vi "Configure General Settings.vi"(1 "Jump Mode":u16(ring) items=["After Repetitions", "As soon as possible"], 2 "Wait Trigger on":u16(ring) items=["First Sample", "Last Sample"], 4 "Burst Selection":u16(ring) items=["Number of Cycles", "Default", "Minimum", "Maximum"], 5 "Burst Count":u32=1, 6 "Run Mode":u16(ring) items=["Continuous", "Single/Burst", "Triggered Continuous", "Stepped", "Advanced"], 7 "error in (no error)":errorcluster, 8 "Sample Decreasing Startegy":u16(ring) items=["Decimation", "Cut Tail", "Cut Head"], 9 "Sample Increasing Startegy":u16(ring) items=["Interpolation", "Return Zero", "Hold Last", "Samples Multiplication"], 10 "VISA resource name":refnum<visa-resource-name>) -> (0 "error out":errorcluster, 3 "VISA resource name out":refnum<visa-resource-name>)   [LabVIEW 2020, in "Active Technologies AWG3000.lvlib"]
uses:
  Active Technologies AWG3000.lvlib
panel:
  # "RESAMPLE STRATEGY"
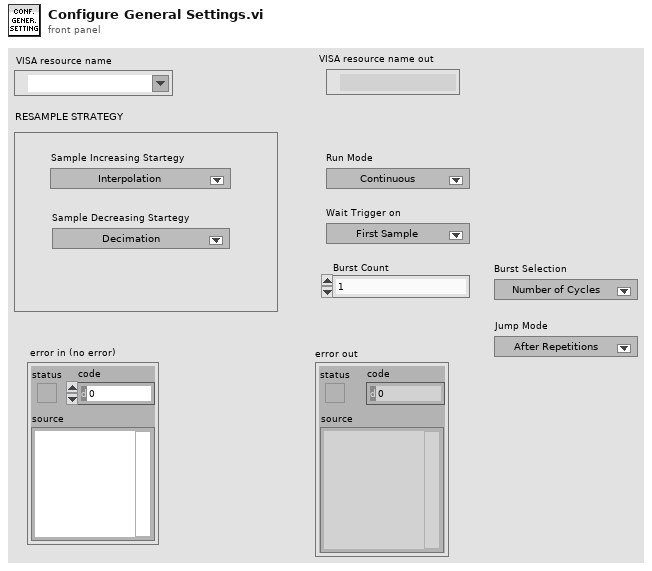
[diagram p1: front panel]
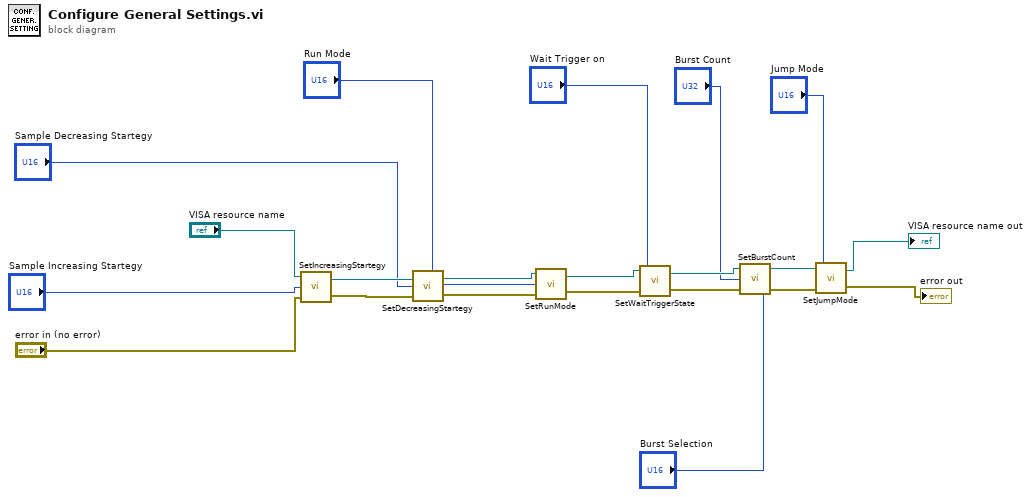
[diagram p0: block diagram]
diagram:
  n1 = call "SetIncreasingStartegy.vi"("error in (no error)"="error in (no error)", "Sample Increasing Startegy"="Sample Increasing Startegy", "VISA resource name"="VISA resource name") -> ("error out"=w16:errorcluster, "VISA resource name out"=w21:refnum<visa-resource-name>)
  n2 = call "SetDecreasingStartegy.vi"("error in (no error)"=w16, "Sample Decreasing Startegy"="Sample Decreasing Startegy", "VISA resource name"=w21) -> ("error out"=w14:errorcluster, "VISA resource name out"=w15:refnum<visa-resource-name>)
  n3 = call "SetRunMode.vi"("error in (no error)"=w14, "Run Mode"="Run Mode", "VISA resource name"=w15) -> ("error out"=w12:errorcluster, "VISA resource name out"=w13:refnum<visa-resource-name>)
  n4 = call "SetWaitTriggerState.vi"("error in (no error)"=w12, "Wait Trigger on"="Wait Trigger on", "VISA resource name"=w13) -> ("error out"=w9:errorcluster, "VISA resource name out"=w10:refnum<visa-resource-name>)
  n5 = call "SetBurstCount.vi"("Burst Selection"="Burst Selection", "error in (no error)"=w9, "Burst Count"="Burst Count", "VISA resource name"=w10) -> ("error out"=w5:errorcluster, "VISA resource name out"=w6:refnum<visa-resource-name>)
  n6 = call "SetJumpMode.vi"("error in (no error)"=w5, "Jump Mode"="Jump Mode", "VISA resource name"=w6) -> ("error out"=→"error out":errorcluster, "VISA resource name out"=→"VISA resource name out":refnum<visa-resource-name>)
